vi "Get all Sub Project Items by Type.vi"(8 "error in (no error)":errorcluster, 10 "Type String":string, 11 "ProjectItem":refnum<vi>) -> (0 "error out":errorcluster, 2 "Project Items":refnum<vi>[](array[refnum]))   [LabVIEW 2020, in "TEST JKI State Machine API.lvlib"]
uses:
  TEST JKI State Machine API.lvlib
panel:
  out "dup ProjectItem":refnum<vi>
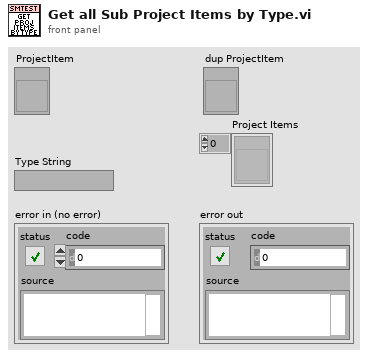
[diagram p1: front panel]
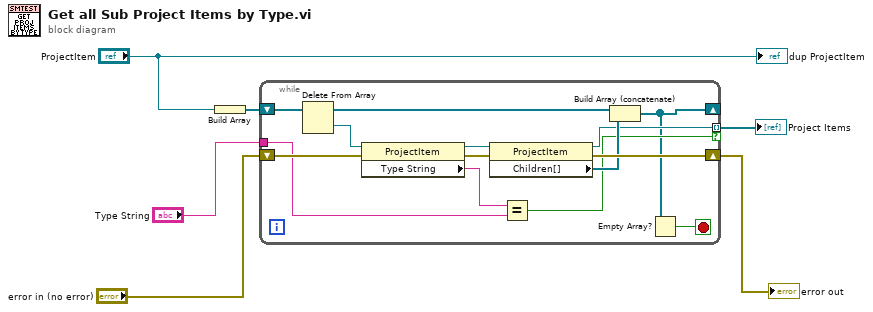
[diagram p0: block diagram]
diagram:
  n1 = Build Array("ProjectItem") -> (w2:refnum<vi>[])
  n2 = while {
    shift-right: [w7] -> _
    shift-left: w2 -> [w17]
    shift-right: [w18] -> w6
    shift-left: "error in (no error)" -> [w13]
    tunnel: "Type String" -> [w11]
    tunnel: [w10] -> w5 mode=indexing if=w9
    stop <- w8 stop-if-true
    n3 = Delete From Array(array=w17) -> (deleted portion=w16:refnum<vi>, array with subset deleted=w15:refnum<vi>[])  [unwired: 2 in]
    n4 = property class="ProjectItem"(reference=w16, error in=w13) -> (reference out=w20:refnum<vi>, error out=w19:errorcluster, "Type String"=w12:string)
    n5 = property class="ProjectItem"(reference=w20, error in=w19) -> (reference out=w10:refnum<vi>, error out=w18:errorcluster, "Children[]"=w14:refnum<vi>[])
    n6 = Equal?(x=w12, y=w11) -> (x = y?=w9:bool)
    n7 = Build Array (concatenate)(w15, w14) -> (w7:refnum<vi>[])
    n8 = Empty Array?(array=w7) -> (empty?=w8:bool)
  }
  "error out" <- w6
  "Project Items" <- w5
  "dup ProjectItem" <- "ProjectItem"
